vi "Create_upload_jlink_file_stm32.vi"(0 ".mot file":path, 7 "path":path, 11 "error in":errorcluster) -> (15 "error out":errorcluster)   [LabVIEW 2023]
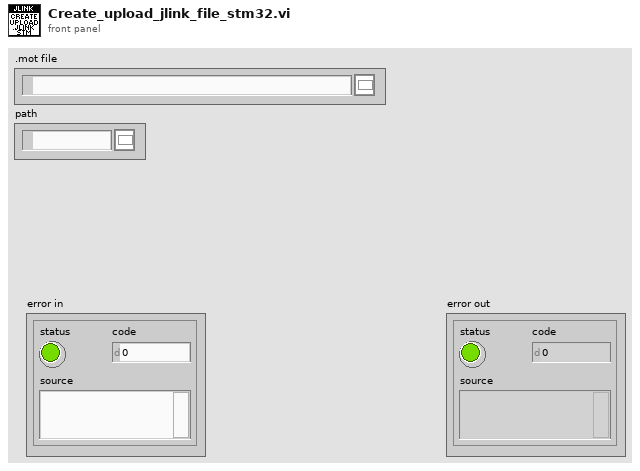
[diagram p1: front panel]
types:
  T1 = enum16{"open", "replace", "create", "open or create", "replace or create", "replace or create with confirmation"}
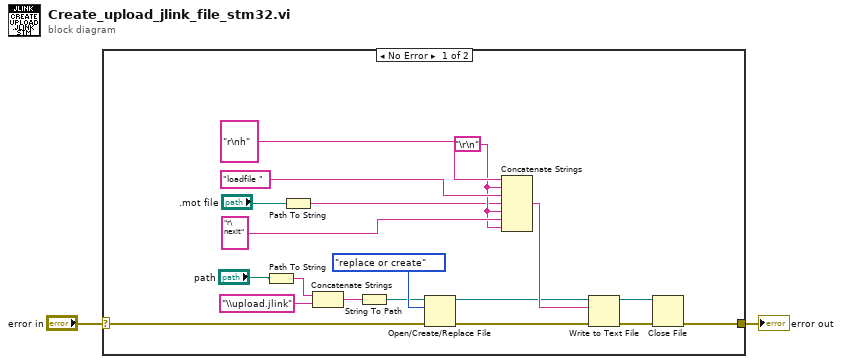
[diagram p0: block diagram]
diagram:
  n1 = case shown="No Error" "error in" {
    selector: "error in" -> [w4 w22]
    tunnel: [w3 w22] -> w1
    frame No Error {
      w16 = "\r\n"
      n2 = Path To String(path="path") -> (string=w7:string)
      n3 = Path To String(path=".mot file") -> (string=w15:string)
      n4 = Concatenate Strings(w7, "\\upload.jlink" ("string")) -> (w8:string)
      n5 = String To Path(string=w8) -> (path=w6:path)
      n6 = Open/Create/Replace File(file path (use dialog)=w6, error in=w4, operation (0:open)=T1."replace or create") -> (refnum out=w13:refnum<file>, error out=w12:errorcluster)  [unwired: 3 in, 1 out]
      n7 = Concatenate Strings("r\nh" ("string"), w16, "loadfile " ("string"), w15, w16, "r\nexit" ("string"), w16) -> (w17:string)
      n8 = Write to Text File(file (use dialog)=w13, text=w17, error in=w12) -> (refnum out=w11:refnum<file>, error out=w10:errorcluster)  [unwired: 1 in, 1 out]
      n9 = Close File(refnum=w11, error in=w10) -> (error out=w3:errorcluster)  [unwired: 1 out]
    }
    frame Error {
    }
  }
  "error out" <- w1
